vi "Test Broadcast Unfiltered Debug Data Log.vi"(8 "error in (no error)":errorcluster, 11 "Test Case In":refnum<class "Debugger Test.lvclass">) -> (0 "error out":errorcluster, 3 "Test Case Out":refnum<class "Debugger Test.lvclass">)   [LabVIEW 2020, in "Debugger Test.lvclass"]
uses:
  Debugger Test.lvclass
  Debugger Test.lvclass/Debugger Test.ctl
  01074fa8-ee8a-411d-bc8b-fc92c4f90959.vi
  source/Process/Debug Process.lvclass
  source/Debugger/Debugger.lvclass
  C:/Users/anton/Documents/GitHub/triarc-debugger/source/Process/Debug Process.lvclass
  source/Debug Data/Debug Data.lvclass
  source/Debug Data/Raw Debug Data.ctl
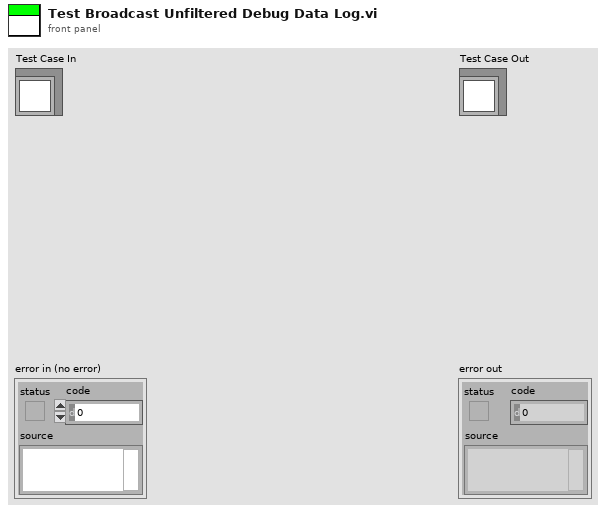
[diagram p1: front panel]
types:
  T1 = typedef "Debug Data.lvclass/Raw Debug Data.ctl" = cluster{"Action":string, "Call Chain":string, "Process":string, "Message":string, "Message Data":variant, "Time":u32}
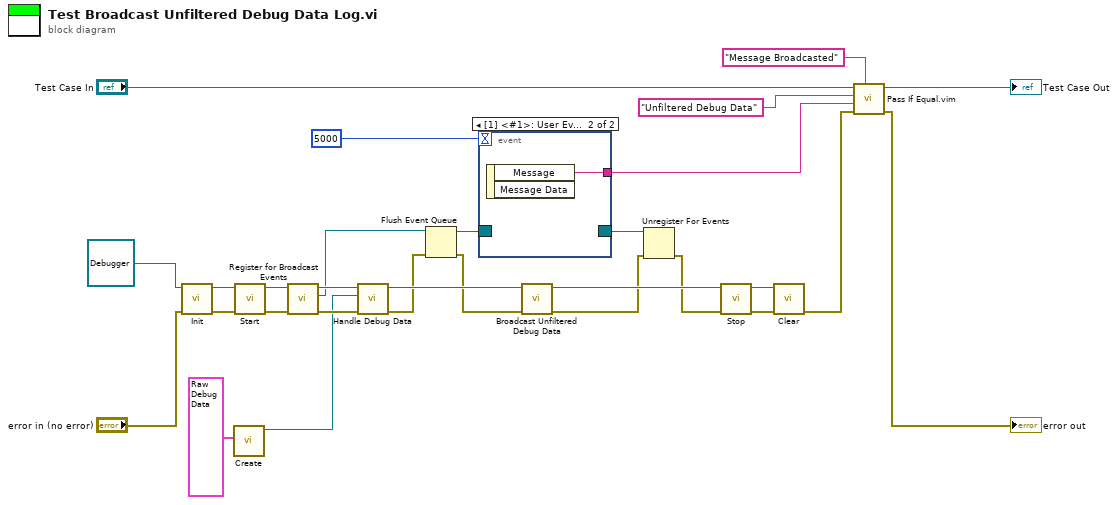
[diagram p0: block diagram]
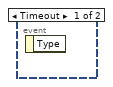
[diagram p2: hidden frame]
diagram:
  n1 = call-dynamic "Init.vi"("error in (no error)"="error in (no error)", "Process In"=refnum<class "Debugger.lvclass"> refnum ("Debug Data Event In 2")) -> ("error out"=w25:errorcluster, "Process Out"=w26:refnum<class "Debugger.lvclass">)  [unwired: 8 in]
  n2 = call "Create.vi"("Debug Data Cluster"=T1 {"Action"="", "Call Chain"="", "Process"="Test", "Message"="", "Message Data"=variant, "Time"=0}) -> ("Debug Data out"=w12:refnum<class "Debug Data.lvclass">)  [unwired: 9 in, 1 out]
  n3 = call "Start.vi"("error in (no error)"=w25, "Process In"=w26) -> ("error out"=w23:errorcluster, "Process Out"=w24:refnum<class "Debugger.lvclass">)  [unwired: 7 in, 1 out]
  n4 = call "Register for Broadcast Events.vi"("error in (no error)"=w23, "Process In"=w24) -> ("error out"=w22:errorcluster, "Event Registration Refnum Out"=w4:refnum<event-registration>, "Process Out"=w16:refnum<class "Debugger.lvclass">)  [unwired: 7 in]
  n5 = call-dynamic "Handle Debug Data.vi"("error in (no error)"=w22, "Debug Data.lvclass"=w12, "Debug Data Event In"=w16) -> ("error out"=w20:errorcluster, "Debug Data Event Out"=w21:refnum<class "Debugger.lvclass">)  [unwired: 7 in]
  n6 = Flush Event Queue(0:w4, 3:w20) -> (8:w3:refnum<event-registration>, 11:w5:errorcluster)  [unwired: 4 in, 1 out]
  n7 = event shown="[1] <#1>: User Event" {
    selector: w3 -> [_ _]
    dyn-events: [_ _] -> w9
    timeout: 5000 -> [_ _]
    tunnel: [_ w30] -> w8
    event Timeout {
      n8 = event-data() -> ()  [unwired: 1 in, 1 out]
    }
    event User Event {
      n9 = event-data() -> ("Message"=w30:string)  [unwired: 1 in, 1 out]
    }
  }
  n10 = call "Broadcast Unfiltered Debug Data.vi"("error in (no error)"=w5, "Debugger in"=w21) -> ("error out"=w2:errorcluster, "Debugger out"=w19:refnum<class "Debugger.lvclass">)  [unwired: 8 in]
  n11 = Unregister For Events(event registration refnum=w9, error in=w2) -> (error out=w1:errorcluster)
  n12 = call "Stop.vi"("error in (no error)"=w1, "Process In"=w19) -> ("error out"=w17:errorcluster, "Process Out"=w18:refnum<class "Debugger.lvclass">)  [unwired: 7 in, 1 out]
  n13 = call-dynamic "Clear.vi"("error in (no error)"=w17, "Process In"=w18) -> ("error out"=w13:errorcluster)  [unwired: 9 in]
  n14 = call "Pass If Equal.vim"("Description"="Message Broadcasted", "error in (no error)"=w13, "Actual"=w8, "Expected"="Unfiltered Debug Data", "LUnit Test Case In"="Test Case In") -> ("error out"=→"error out":errorcluster, "LUnit Test Case Out"=→"Test Case Out":refnum<class "Debugger Test.lvclass">)  [unwired: 5 in]
